vi "c ctre phoenixpro set configs.vi"(0 "context":u32(ring) items=["ContextAPI", "ContextDiagServer"], 1 "values":string, 2 "futureProofConfigs":bool, 3 "useDid":bool, 5 "network":string, 7 "deviceHash":i32, 9 "timeoutSeconds":dbl, 11 "error in (no error)":errorcluster, 12 "value_len":u32, 13 "overrideIfDuplicate":bool) -> (4 "function return":i32, 15 "error out":errorcluster)   [LabVIEW 2020, in "CTRE_PhoenixTools.lvlib"]
doc: "CTREXPORT int c_ctre_phoenixpro_set_configs(\n Context context,\n const char *network,\n int deviceHash,\n double timeoutSeconds,\n const char *values,\n uint32_t value_len,\n bool futureProofConfigs,\n bool overrideIfDuplicate,\n bool useDid);"
uses:
  CTRE_PhoenixTools.lvlib
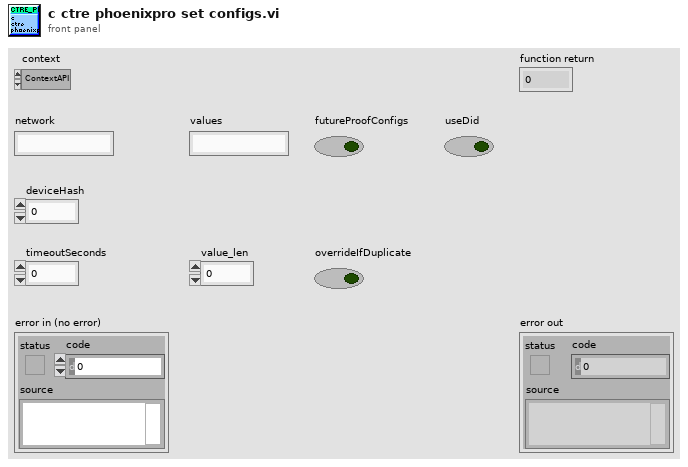
[diagram p1: front panel]
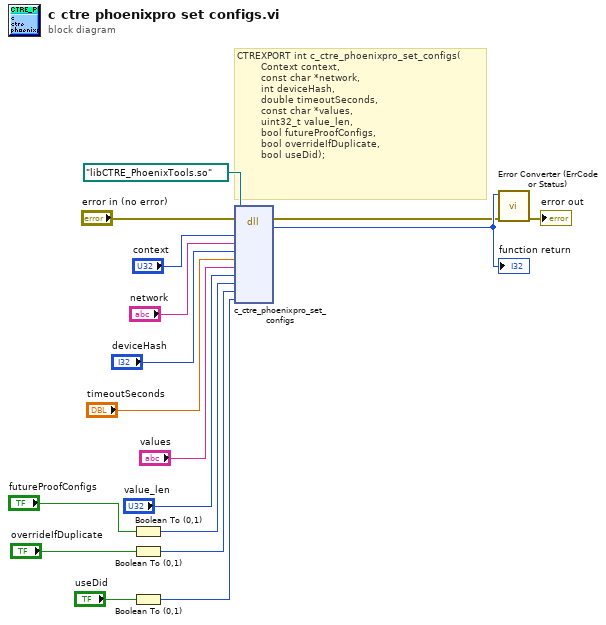
[diagram p0: block diagram]
diagram:
  # "CTREXPORT int c_ctre_phoenixpro_set_configs(\n        Context context,\n        const char *network,\n        int deviceHash,\n        double timeoutSeconds,\n        const char *values,\n        uint32_t value_len,\n        bool futureProofConfigs,\n        bool overrideIfDuplicate,\n        bool useDid);"
  n1 = Boolean To (0,1)(Boolean="futureProofConfigs") -> (0, 1=w9:i16)
  n2 = Boolean To (0,1)(Boolean="overrideIfDuplicate") -> (0, 1=w7:i16)
  n3 = Boolean To (0,1)(Boolean="useDid") -> (0, 1=w5:i16)
  n4 = dll-call lib="?" fn="c_ctre_phoenixpro_set_configs"(path in=path "libCTRE_PhoenixTools.so", error in="error in (no error)", "context"="context", "network"="network", "deviceHash"="deviceHash", "timeoutSeconds"="timeoutSeconds", "values"="values", "value_len"="value_len", "futureProofConfigs"=w9, "overrideIfDuplicate"=w7, "useDid"=w5) -> (error out=w3:errorcluster, w17:i32)  [unwired: 10 in, 1 out]
  "function return" <- w17
  n5 = call "Error Converter (ErrCode or Status).vi"("error in (no error)"=w3, "error code"=w17) -> ("error out"=→"error out":errorcluster)  [unwired: 9 in]
